vi "ASCII 쓰기.vi"() -> ()   [LabVIEW 2014]
panel:
  in  "파일 경로(대화 상자 사용)":path
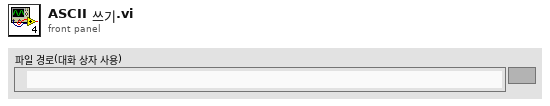
[diagram p1: front panel]
types:
  T1 = enum16{"open", "replace", "create", "open or create", "replace or create", "replace or create with confirmation"}
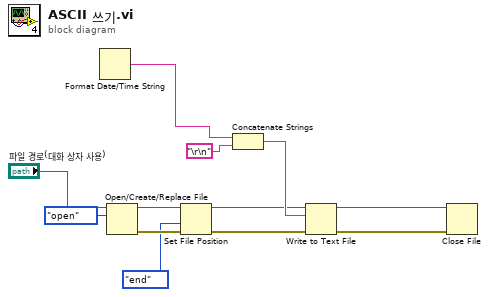
[diagram p0: block diagram]
diagram:
  n1 = Format Date/Time String() -> (date/time string=w7:string)  [unwired: 3 in]
  n2 = Open/Create/Replace File(file path (use dialog)="파일 경로(대화 상자 사용)", operation (0:open)=T1."open" ("동작(0:open)")) -> (refnum out=w6:refnum<file>, error out=w5:errorcluster)  [unwired: 4 in, 1 out]
  n3 = Set File Position(refnum=w6, from (0:start)=enum16{"start", "end", "current"}."end" ("시작(0:시작)"), error in=w5) -> (refnum out=w3:refnum<file>, error out=w2:errorcluster)  [unwired: 1 in]
  n4 = Concatenate Strings(w7, "\r\n") -> (w9:string)
  n5 = Write to Text File(file (use dialog)=w3, text=w9, error in=w2) -> (refnum out=w12:refnum<file>, error out=w11:errorcluster)  [unwired: 1 in, 1 out]
  n6 = Close File(refnum=w12, error in=w11) -> ()  [unwired: 2 out]
